vi "Add Tests.vi"(8 "error in (no error)":errorcluster, 10 "Tests":string[](array[string]), 11 "Result Model by Reference In":refnum<class "Result Model by Reference.lvclass">) -> (0 "error out":errorcluster)   [LabVIEW 2020, in "Result Model by Reference.lvclass"]
uses:
  Result Model by Reference.lvclass
  Result Model/Result Model.lvclass
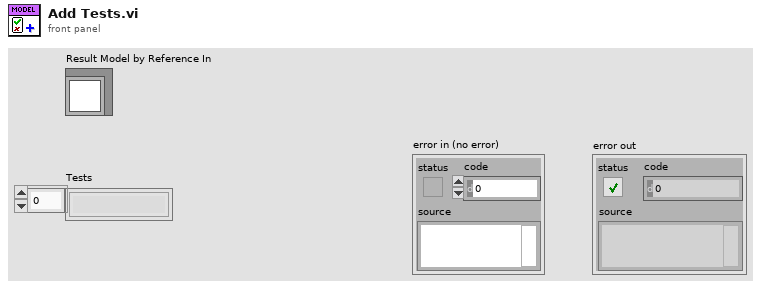
[diagram p1: front panel]
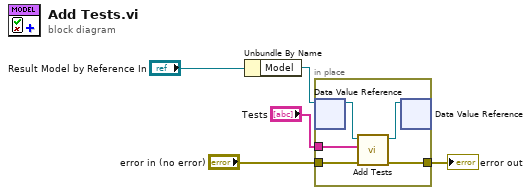
[diagram p0: block diagram]
diagram:
  n1 = Unbundle By Name("Result Model by Reference In") -> ("Model"=w5:refnum<data-value>)
  n2 = in-place {
    in-place-border: "error in (no error)" -> [w10]
    in-place-border: [w9] -> w1
    in-place-border: "Tests" -> [w6]
    n3 = in-place-dvr #1(w5) -> (w7:refnum<class "Result Model.lvclass">)  [unwired: 1 out]
    n4 = call "Add Tests.vi"("error in (no error)"=w10, "Tests"=w6, "Result Model In"=w7) -> ("error out"=w9:errorcluster, "Result Model Out"=w8:refnum<class "Result Model.lvclass">)  [unwired: 7 in]
    n5 = in-place-dvr #1(w8) -> ()  [unwired: 2 out]
  }
  "error out" <- w1
